vi "Ritter Rate Average.vi"(6 "Avg Interval (Sec)":i32, 8 "Error In":errorcluster, 9 "Totalized Flow (cuft)":dbl, 11 "Array IN":dbl[](array[numeric])) -> (0 "Error Out":errorcluster, 2 "Average (BTU/HR) (Out)":dbl, 3 "Array OUT":dbl[](array[numeric]))   [LabVIEW 2023]
panel:
  out "Individual Flow Rates (cuft/sec)":dbl[](array[numeric])
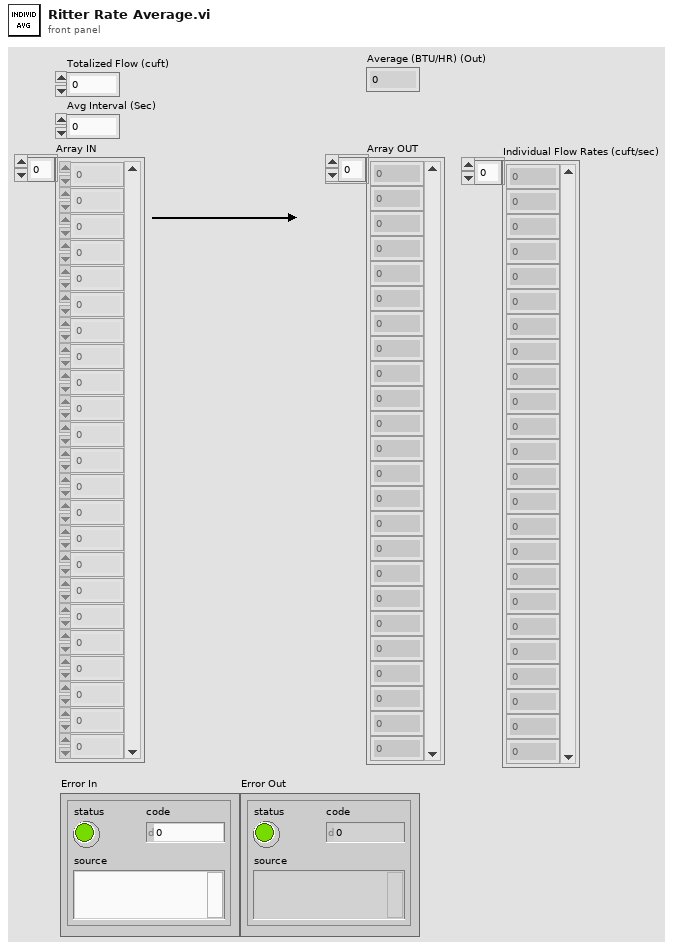
[diagram p1: front panel]
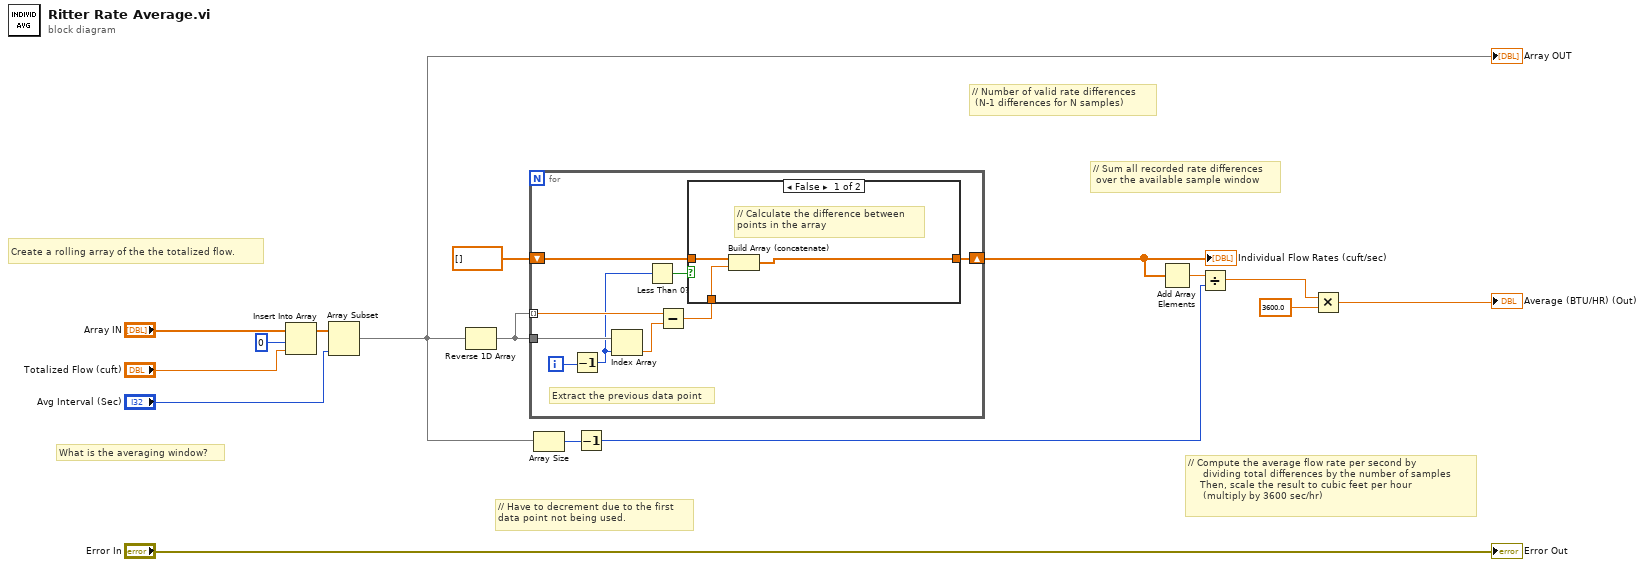
[diagram p0: block diagram]
diagram:
  # "// Compute the average flow rate per second by\n     dividing total differences by the number of samples\n    Then, scale the result to cubic feet per hour\n     (multiply by 3600 sec/hr)"
  # "// Sum all recorded rate differences\n over the available sample window"
  # "What is the averaging window?"
  # "// Number of valid rate differences\n (N-1 differences for N samples)"
  # "// Have to decrement due to the first\ndata point not being used."
  # "Create a rolling array of the the totalized flow."
  n1 = Insert Into Array(array="Array IN", index=0, new element="Totalized Flow (cuft)") -> (w15:dbl[])
  n2 = Array Subset(array=w15, length="Avg Interval (Sec)") -> (w11:dbl[])  [unwired: 1 in]
  "Array OUT" <- w11
  n3 = Reverse 1D Array(array=w11) -> (reversed array=w10:dbl[])
  n4 = for {
    tunnel: w10 -> [w25] mode=indexing
    tunnel: w10 -> [w24]
    shift-right: [w19] -> w6
    shift-left: dbl[] [] -> [w21]
    i -> [w22]
    # "Extract the previous data point"
    n5 = Decrement(x=w22) -> (x-1=w18:i32)
    n6 = Index Array(array=w24, index=w18) -> (element=w23:dbl)
    n7 = Less Than 0?(x=w18) -> (x < 0?=w17:bool)
    n8 = Subtract(x=w25, y=w23) -> (x-y=w20:dbl)
    n9 = case shown="False" w17 {
      tunnel: w21 -> [w28 w29]
      tunnel: w20 -> [w27 _]
      tunnel: [w26 w29] -> w19
      frame False {
        # "// Calculate the difference between\npoints in the array"
        n10 = Build Array (concatenate)(w28, w27) -> (w26:dbl[])
      }
      frame True {
        # "// The first reading alone is insufficient\n      because we need a difference."
      }
    }
  }
  "Individual Flow Rates (cuft/sec)" <- w6
  n11 = Array Size(array=w11) -> (size(s)=w9:i32)
  n12 = Decrement(x=w9) -> (x-1=w8:i32)
  n13 = Add Array Elements(numeric array=w6) -> (sum=w3:dbl)
  n14 = Divide(x=w3, y=w8) -> (x/y=w2:dbl)
  n15 = Multiply(x=w2, y=3600.0) -> (x*y=→"Average (BTU/HR) (Out)":dbl)
  "Error Out" <- "Error In"
